vi "insert_into_log.vi"(5 "data_type":T1, 6 "offset_from_bof":u32, 7 "dims":T2, 8 "error in (no error)":errorcluster, 9 "Location":string, 10 "Data":variant, 11 "raw_stream_logger in":refnum<class "raw_stream_logger.lvclass">) -> (0 "error out":errorcluster, 3 "raw_stream_logger out":refnum<class "raw_stream_logger.lvclass">)   [LabVIEW 2015, in "raw_stream_logger.lvclass"]
uses:
  raw_stream_logger.lvclass
  Data Logger Class/data_dimensionality.ctl
  Data Logger Class/logger_data_types.ctl
  raw_stream_logger.lvclass/raw_stream_logger.ctl
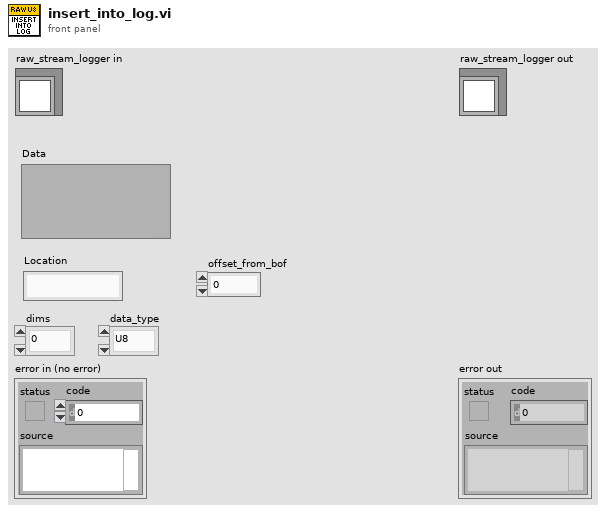
[diagram p1: front panel]
types:
  T1 = typedef "logger_data_types.ctl" = enum16{"U8", "I8", "U16", "I16", "U32", "I32", "DBL", "String"}
  T2 = typedef "data_dimensionality.ctl" = enum16{"0", "1", "2"}
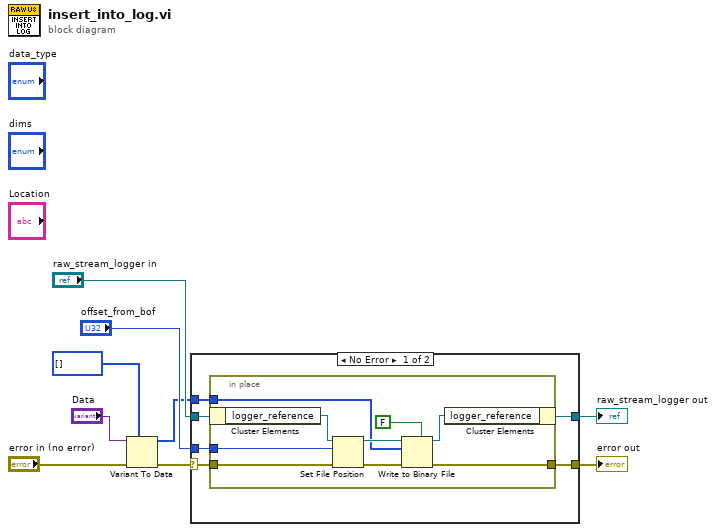
[diagram p0: block diagram]
diagram:
  n1 = Variant To Data(error in="error in (no error)", type=u8[] [], Variant="Data") -> (data=w5:u8[], error out=w1:errorcluster)
  n2 = case shown="No Error" w1 {
    selector: w1 -> [w13 w26]
    tunnel: "raw_stream_logger in" -> [w15 w25]
    tunnel: "offset_from_bof" -> [w14 _]
    tunnel: w5 -> [w12 _]
    tunnel: [w11 w25] -> w4
    tunnel: [w10 w26] -> w3
    frame No Error {
      n3 = in-place {
        in-place-border: w14 -> [w23]
        in-place-border: w13 -> [w22]
        in-place-border: w12 -> [w20]
        in-place-border: [w16] -> w10
        n4 = in-place-cluster #1(w15) -> ("logger_reference"=w24:refnum<file>)
        n5 = Set File Position(offset (in bytes) (0)=w23, refnum=w24, error in=w22) -> (refnum out=w21:refnum<file>, error out=w19:errorcluster)  [unwired: 1 in]
        n6 = Write to Binary File(file (use dialog)=w21, data=w20, error in=w19, 5:FALSE ("prepend array or string size? (T)")) -> (refnum out=w17:refnum<file>, error out=w16:errorcluster)  [unwired: 2 in, 1 out]
        n7 = in-place-cluster #1("logger_reference"=w17) -> (w11:refnum<class "raw_stream_logger.lvclass">)
      }
    }
    frame Error {
    }
  }
  "error out" <- w3
  "raw_stream_logger out" <- w4
